vi "NanonisFrame-Demod.vi"(0 "x":dbl, 1 "z":dbl, 2 "Signal":u16(ring) items=["Z Val", "Demod"]) -> (8 "X Out":dbl, 10 "Z Out":dbl, 12 "Speed":dbl, 14 "FO X":dbl, 15 "FO Z":dbl, 16 "FW":dbl, 17 "FH":dbl, 19 "CVAL (nA)":dbl)   [LabVIEW 2017]
uses:
  Program Files/National Instruments/LabVIEW 2019/user.lib/Nanonis Prog Interface V5/Nanonis Prog Interface.lvlib
panel:
  out "Signal value":sgl format="%#_6p"
  out "Signals Names":string[](array[string])
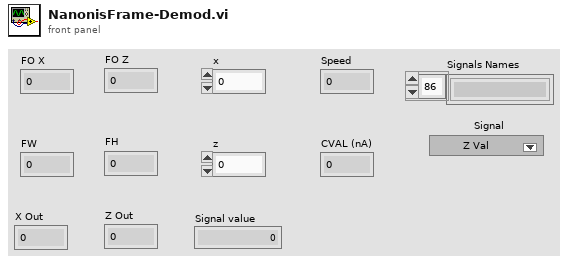
[diagram p1: front panel]
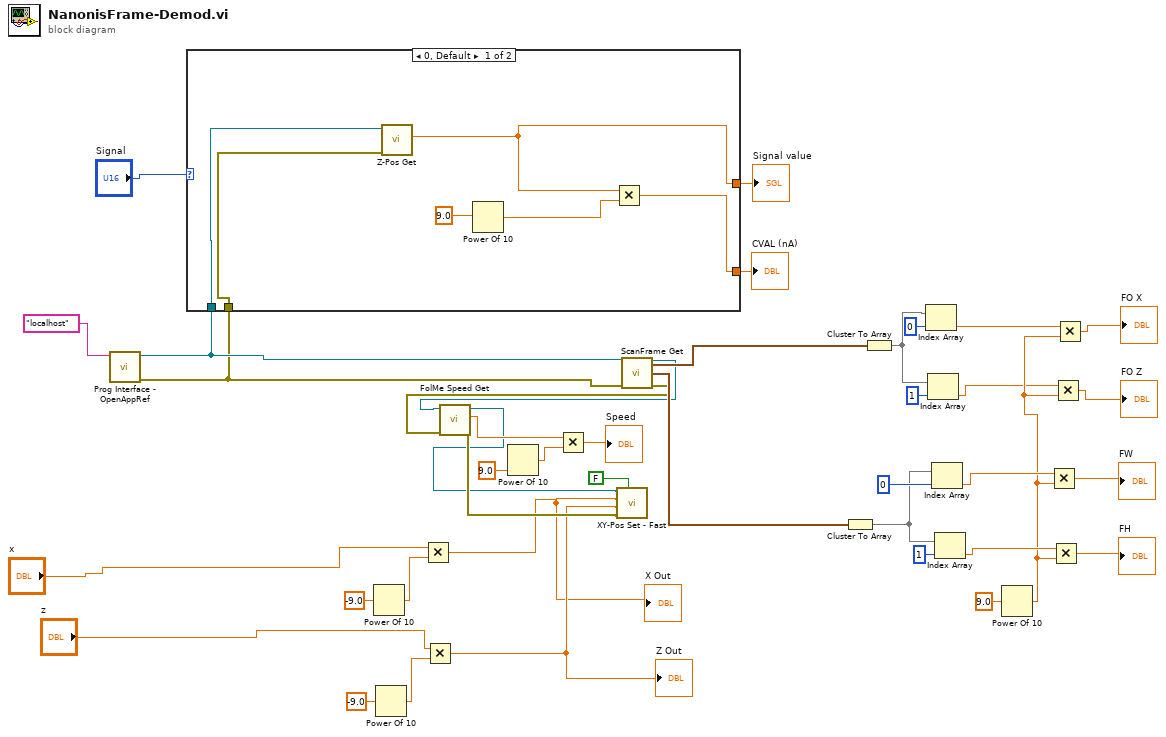
[diagram p0: block diagram]
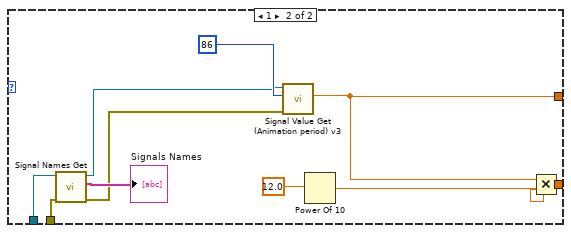
[diagram p2: hidden frame]
diagram:
  n1 = call <userlib>:"Prog Interface - OpenAppRef.vi"("Machine name (local machine IP)"="localhost") -> ("Error out"=w3:errorcluster, "Application reference"=w4:refnum<vi>)  [unwired: 5 in]
  n2 = case shown="0, Default" "Signal" {
    tunnel: [w45 w55] -> w10
    tunnel: w4 -> [w43 w53]
    tunnel: w3 -> [w42 w52]
    tunnel: [w44 w48] -> w2
    frame 0, Default {
      n3 = call <userlib>:"Z-Pos Get.vi"("error in (no error)"=w42, "Application ref in"=w43) -> ("Z position (m)"=w44:sgl)  [unwired: 7 in, 2 out]
      n4 = Power Of 10(x=9.0) -> (10^x=w47:dbl)
      n5 = Multiply(x=w44, y=w47) -> (x*y=w45:dbl)
    }
    frame 1 {
      n6 = call <userlib>:"Signal Names Get.vi"("error in (no error)"=w52, "Application ref in"=w53) -> ("error out"=w50:errorcluster, "Signals Names"=→"Signals Names":string[], "Application ref out"=w49:refnum<vi>)  [unwired: 5 in]
      n7 = call <userlib>:"Signal Value Get (Animation period) v3.vi"("error in (no error)"=w50, "Signal index (0-127)"=i8 86, "Application ref in"=w49) -> ("Signal value"=w48:sgl)  [unwired: 5 in, 2 out]
      n8 = Power Of 10(x=12.0) -> (10^x=w56:dbl)
      n9 = Multiply(x=w48, y=w56) -> (x*y=w55:dbl)
    }
  }
  "CVAL (nA)" <- w10
  "Signal value" <- w2
  n10 = Power Of 10(x=-9.0) -> (10^x=w21:dbl)
  n11 = Power Of 10(x=-9.0) -> (10^x=w19:dbl)
  n12 = Multiply(x="x", y=w21) -> (x*y=w7:dbl)
  "X Out" <- w7
  n13 = Multiply(x="z", y=w19) -> (x*y=w8:dbl)
  "Z Out" <- w8
  n14 = Power Of 10(x=9.0) -> (10^x=w24:dbl)
  n15 = call <userlib>:"ScanFrame Get.vi"("Application ref in"=w4, "error in (no error)"=w3) -> ("Application ref out"=w26:refnum<vi>, "Center coordinates (m)"=w40:cluster{"Xc":sgl, "Yc":sgl}, "Size (m)"=w36:cluster{"Width":sgl, "Height":sgl}, "error out"=w17:errorcluster)  [unwired: 9 in, 1 out]
  n16 = call <userlib>:"FolMe Speed Get.vi"("error in (no error)"=w17, "Application ref in"=w26) -> ("error out"=w9:errorcluster, "Speed (m/s)"=w23:sgl, "Application ref out"=w6:refnum<vi>)  [unwired: 4 in, 1 out]
  n17 = Multiply(x=w23, y=w24) -> (x*y=→"Speed":dbl)
  n18 = call <userlib>:"XY-Pos Set - Fast.vi"("Wait end-of-motion (T=True)"=FALSE, "error in (no error)"=w9, "Y (m)"=w8, "X (m)"=w7, "Application ref in"=w6) -> ()  [unwired: 4 in, 2 out]
  n19 = Cluster To Array(cluster=w36) -> (array=w33:sgl[])
  n20 = Cluster To Array(cluster=w40) -> (array=w39:sgl[])
  n21 = Index Array(array=w39, index=0) -> (element=w14:sgl)
  n22 = Index Array(array=w39, index=1) -> (element=w13:sgl)
  n23 = Index Array(array=w33, index=0) -> (element=w32:sgl)
  n24 = Index Array(array=w33, index=1) -> (element=w31:sgl)
  n25 = Power Of 10(x=9.0) -> (10^x=w29:dbl)
  n26 = Multiply(x=w32, y=w29) -> (x*y=→"FW":dbl)
  n27 = Multiply(x=w31, y=w29) -> (x*y=→"FH":dbl)
  n28 = Multiply(x=w13, y=w29) -> (x*y=→"FO Z":dbl)
  n29 = Multiply(x=w14, y=w29) -> (x*y=→"FO X":dbl)
